vi "Find Keepers.vi"(10 "Support Map":map{i32, set{i32}}(c390), 11 "Brick Map":map{i32, T1[]}(c390)) -> (2 "Potential Remove Out":i32[](array[numeric]), 3 "Keep Array Out":i32[](array[numeric]))   [LabVIEW 2023]
uses:
  Cluster_Node.ctl
  <vilib>/Utility/miscctls.llb/LVMapReplaceAction.ctl
panel:
  out "Keep Map":map{i32, bool}(c390)
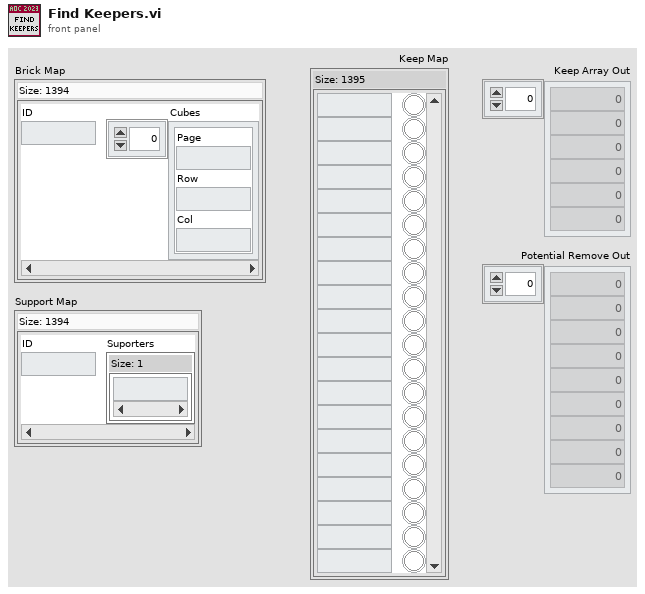
[diagram p1: front panel]
types:
  T1 = typedef "Cluster_Node.ctl" = cluster{"Page":i32, "Row":i32, "Col":i32}
  T2 = typedef "LVMapReplaceAction.ctl" = enum32{"Modify Entry only if found", "Add or Modify Entry", "Delete Entry"}
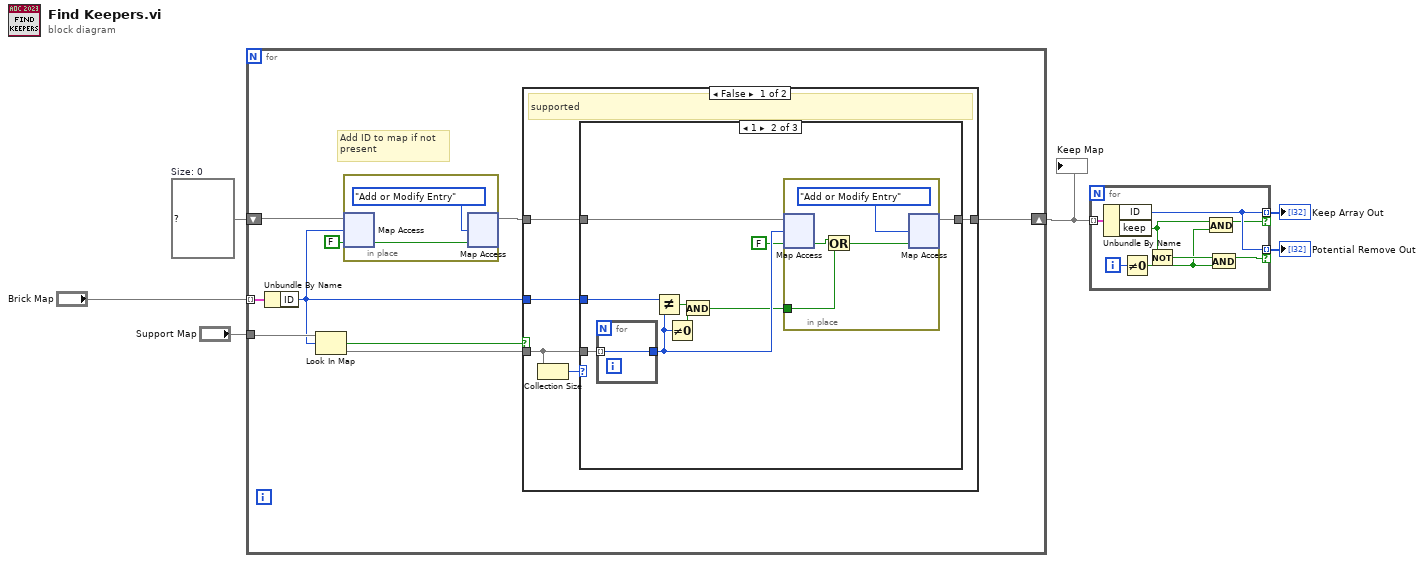
[diagram p0: block diagram]
diagram:
  w4 = map{i32, bool} {}  # Size: 0
  n1 = for {
    tunnel: "Brick Map" -> [w15] mode=indexing
    tunnel: "Support Map" -> [w14]
    shift-right: [w13] -> w3
    shift-left: w4 -> [w12]
    # "Add ID to map if not\npresent"
    n2 = Unbundle By Name(w15) -> ("ID"=w11:i32)
    n3 = Look In Map(map=w14, key=w11) -> (key not found?=w10:bool, value=w9:set{i32})  [unwired: 1 in]
    n4 = in-place {
      n5 = in-place-map #1(w12, w11, FALSE ("keep")) -> (w16:bool)  [unwired: 1 out]
      n6 = in-place-map #1(w16, LVMapReplaceAction."Add or Modify Entry" ("action")) -> (w8:map{i32, bool})  [unwired: 2 out]
    }
    n7 = case shown="False" w10 {
      tunnel: w9 -> [w21 _]
      tunnel: w8 -> [w20 w39]
      tunnel: w11 -> [w19 _]
      tunnel: [w18 w39] -> w13
      frame False {
        # "supported"
        n8 = Collection Size(1:w21) -> (0:w22:i32)
        n9 = case shown="1" w22 {
          tunnel: w21 -> [_ w32 _]
          tunnel: w20 -> [w23 w31 w38]
          tunnel: w19 -> [_ w29 _]
          tunnel: [w23 w30 w38] -> w18
          frame ..0 {
            # "Never supoosed to happen"
            # "every ID should have support"
          }
          frame 1 {
            n10 = for {
              tunnel: w32 -> [w37] mode=indexing
              tunnel: [w37] -> w28
            }
            n11 = Not Equal?(x=w29, y=w28) -> (x != y?=w27:bool)
            n12 = Not Equal To 0?(x=w28) -> (x != 0?=w26:bool)
            n13 = And(x=w27, y=w26) -> (x .and. y?=w24:bool)
            n14 = in-place {
              in-place-border: w24 -> [w34]
              n15 = in-place-map #2(w31, w28, FALSE ("keep")) -> (w35:bool)  [unwired: 1 out]
              n16 = Or(x=w35, y=w34) -> (x .or. y?=w33:bool)
              n17 = in-place-map #2(w33, LVMapReplaceAction."Add or Modify Entry" ("action")) -> (w30:map{i32, bool})  [unwired: 2 out]
            }
          }
          frame 2.. {
            # "Has multiple supporters"
          }
        }
      }
      frame True {
        # "All should be supported \nso this should never happen"
        # "not supported"
      }
    }
  }
  "Keep Map" <- w3
  n18 = for {
    tunnel: w3 -> [w47] mode=indexing
    tunnel: [w46] -> w2 mode=indexing if=w42
    tunnel: [w46] -> w1 mode=indexing if=w43
    i -> [w41]
    n19 = Unbundle By Name(w47) -> ("ID"=w46:i32, "keep"=w45:bool)
    n20 = Not Equal To 0?(x=w41) -> (x != 0?=w40:bool)
    n21 = Not(x=w45) -> (.not. x?=w44:bool)
    n22 = And(x=w45, y=w40) -> (x .and. y?=w42:bool)
    n23 = And(x=w44, y=w40) -> (x .and. y?=w43:bool)
  }
  "Keep Array Out" <- w2
  "Potential Remove Out" <- w1
